vi "getSVP.vi"(4 "Progress":refnum<vi>, 5 "vol":sgl[][][](array[numeric]), 6 "OCT filename":string, 7 "Output Path":path) -> (1 "SVP":u16[][](array[numeric]))   [LabVIEW 2017]
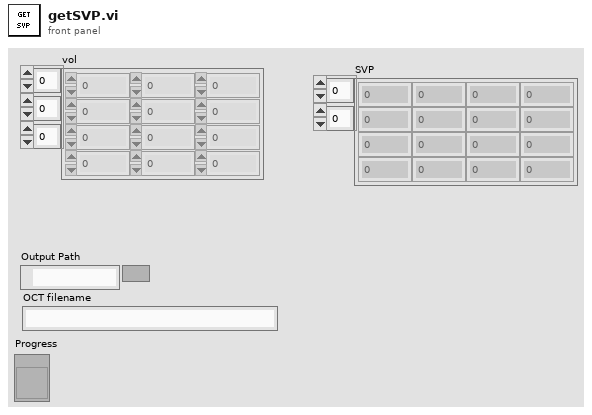
[diagram p1: front panel]
types:
  T1 = typedef "Image Type" = u32
  T2 = typedef "IMAQ Image.ctl" = refnum<image>
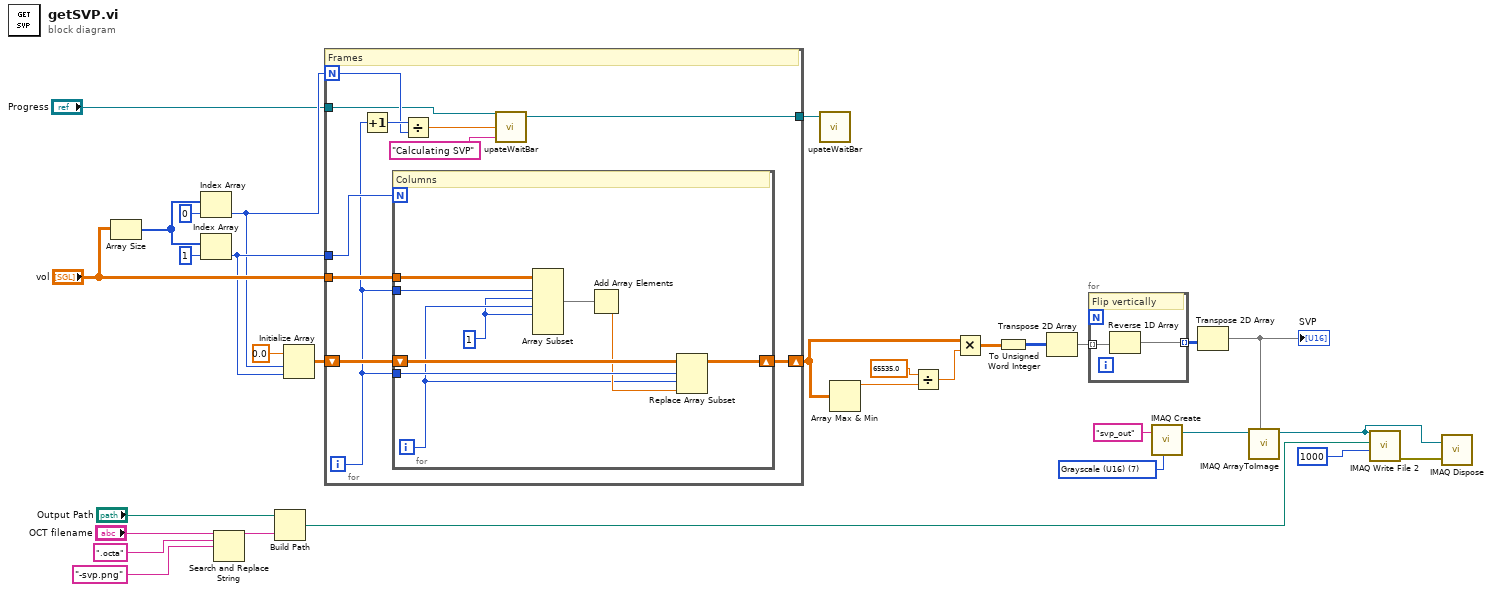
[diagram p0: block diagram]
diagram:
  w11 = T1 7 items=["Grayscale (U8)", "Grayscale (I16)", "Grayscale (SGL)", "Complex (CSG)", "RGB (U32)", "HSL (U32)", "RGB (U64)", "Grayscale (U16)"] ("Image Type")
  n1 = Array Size(array="vol") -> (size(s)=w29:i32[])
  n2 = Index Array(array=w29, index=0) -> (element=w25:i32)
  n3 = Index Array(array=w29, index=1) -> (element=w26:i32)
  n4 = Search and Replace String(input string="OCT filename", search string=".octa", replace string="-svp.png" ("replace string (\"\")")) -> (result string=w15:string)  [unwired: 5 in, 3 out]
  n5 = Build Path(base path="Output Path", name or relative path=w15) -> (appended path=w13:path)
  n6 = Initialize Array(sgl 0.0 ("element"), w25, w26) -> (w24:sgl[][])
  n7 = for {
    N: w25 -> [w36]
    tunnel: "vol" -> [w42]
    tunnel: w26 -> [w41]
    shift-right: [w39] -> w21
    shift-left: w24 -> [w40]
    tunnel: "Progress" -> [w34]
    tunnel: [w32] -> w1
    i -> [w38]
    # "Frames"
    n8 = Increment(x=w38) -> (x+1=w37:i32)
    n9 = for {
      N: w41 -> [_]
      tunnel: w42 -> [w51]
      tunnel: w38 -> [w45]
      tunnel: w38 -> [w48]
      shift-right: [w46] -> w39
      shift-left: w40 -> [w49]
      i -> [w44]
      w43 = 1
      # "Columns"
      n10 = Array Subset(array=w51, index (dim 0)=w45, length (dim 0)=w43, index (dim 1)=w44, length (dim 1)=w43) -> (w50:sgl[][][])  [unwired: 2 in]
      n11 = Add Array Elements(numeric array=w50) -> (sum=w47:sgl)
      n12 = Replace Array Subset(array=w49, new element=w47, index (row)=w48, index (col)=w44) -> (w46:sgl[][])
    }
    n13 = Divide(x=w37, y=w36) -> (x/y=w35:dbl)
    n14 = call "upateWaitBar.vi"("waitbar text"="Calculating SVP", "waitbar value [0,1]"=w35, "Progress"=w34) -> ("Updated Progress"=w32:refnum<vi>)  [unwired: 2 in]
  }
  n15 = call "upateWaitBar.vi"("Progress"=w1) -> ()  [unwired: 4 in, 1 out]
  n16 = Array Max & Min(array=w21) -> (max value=w23:sgl)  [unwired: 3 out]
  n17 = Divide(x=sgl 65535.0, y=w23) -> (x/y=w20:sgl)
  n18 = Multiply(x=w21, y=w20) -> (x*y=w19:sgl[][])
  n19 = To Unsigned Word Integer(number=w19) -> (unsigned 16bit integer=w8:u16[][])
  n20 = Transpose 2D Array(2D array=w8) -> (transposed array=w7:u16[][])
  n21 = for {
    tunnel: w7 -> [w53] mode=indexing
    tunnel: [w52] -> w6 mode=indexing
    # "Flip vertically"
    n22 = Reverse 1D Array(array=w53) -> (reversed array=w52:u16[])
  }
  n23 = call "IMAQ Create"("Image Name"="svp_out", "Image Type"=w11) -> ("New Image"=w10:T2)  [unwired: 3 in, 1 out]
  n24 = Transpose 2D Array(2D array=w6) -> (transposed array=w5:u16[][])
  "SVP" <- w5
  n25 = call "IMAQ ArrayToImage"("Image Pixels (U16)"=w5, "Image"=w10) -> ("Image Out"=w4:T2)  [unwired: 8 in, 1 out]
  n26 = call-poly "IMAQ Write File 2"("Image Quality"=u32 1000, "File Path"=w13, "Image"=w4) -> ("error out"=w3:errorcluster)  [unwired: 7 in, 1 out]
  n27 = call "IMAQ Dispose"("Image"=w4, "error in (no error)"=w3) -> ()  [unwired: 4 in, 1 out]
